vi "JSON to CBOR.vi"(8 "error in (no error)":errorcluster, 11 "JSON Object":string) -> (0 "error out":errorcluster, 3 "CBOR Hex":string)   [LabVIEW 2020, in "CBOR.lvlib"]
uses:
  CBOR.lvlib
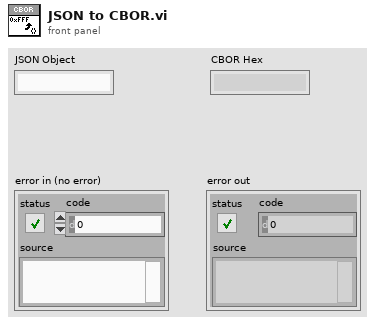
[diagram p1: front panel]
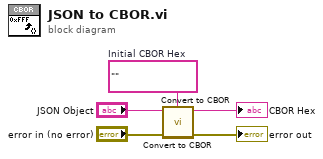
[diagram p0: block diagram]
diagram:
  w1 = ""  # Initial CBOR Hex
  n1 = call "Convert to CBOR.vi"("error in (no error)"="error in (no error)", "CBOR HEX (empty)"=w1, "JSON Object"="JSON Object") -> ("error out"=→"error out":errorcluster, "CBOR HEX"=→"CBOR Hex":string)  [unwired: 7 in]
  n2 = call "Convert to CBOR.vi"() -> ()  [unwired: 10 in, 2 out]
